vi "Initialize Amplitudes.vi"(0 "ToneCloud in":refnum<class "Tone Cloud.lvclass">, 5 "Level in":refnum<class "Level.lvclass">, 11 "error in (no error)":errorcluster) -> (4 "ToneCloud out":refnum<class "Tone Cloud.lvclass">, 15 "error out":errorcluster)   [LabVIEW 2020, in "Tone Cloud.lvclass"]
uses:
  Tone Cloud.lvclass
  Level/Level.lvclass
  Tone Cloud.lvclass/Tone Cloud.ctl
  Level/Level.lvclass/Level.ctl
  ce9a4e56-d8d9-4718-afa1-4568970c8e29.vi
  67dd2368-12ba-4959-8d3f-8fbbdd4b7264.vi
  595b4ae7-b8f7-4111-8c63-d399af629c05.vi
  Level/Read Units.vi
  Utility VIs/Math VIs/interp1 (2D).vi
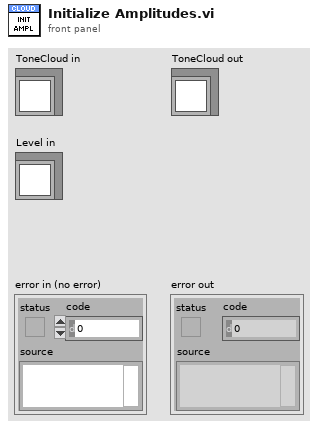
[diagram p1: front panel]
types:
  T1 = typedef "Level.lvclass/LevelUnits.ctl" = enum16{"dB atten", "dB SPL", "dB Vrms", "Volts", "dB mW", "mW", "dB HL", "dB SL"}
  T2 = typedef "Tone Cloud.lvclass/Level Mode.ctl" = enum16{"per component", "total rms"}
  T3 = cluster{"Freq (Hz)":dbl[], "Mag (dB SPL)":dbl[], "Phase (deg)":dbl[]}
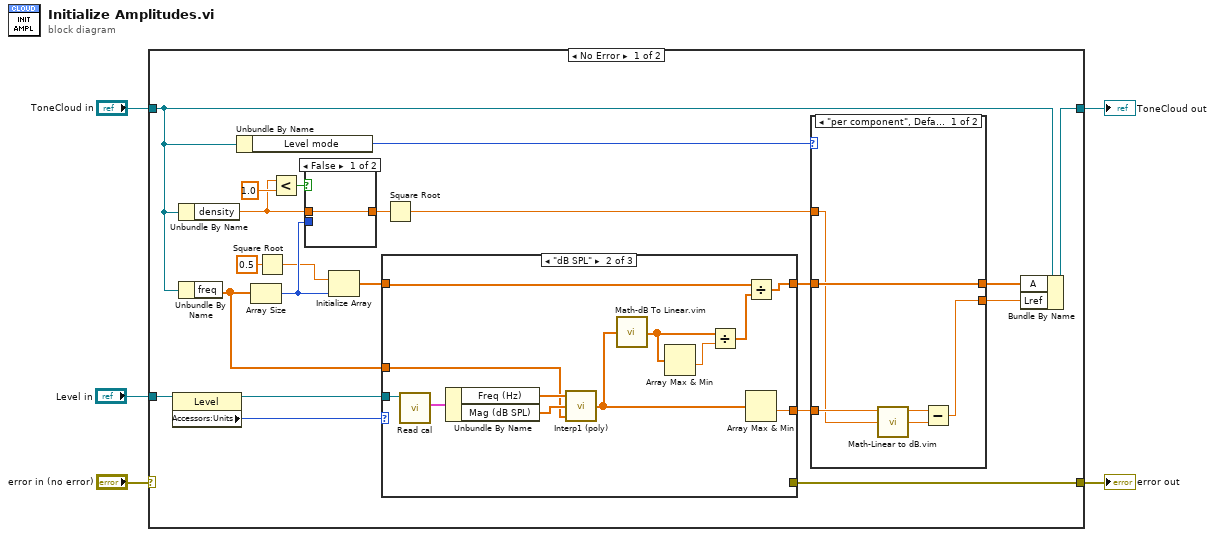
[diagram p0: block diagram]
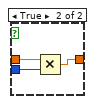
[diagram p2: hidden frame]
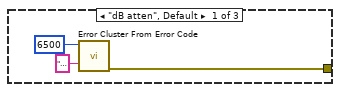
[diagram p3: hidden frame]
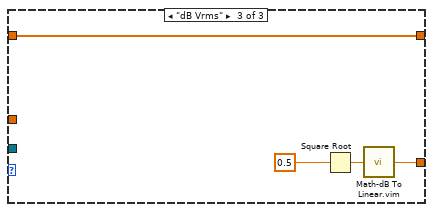
[diagram p4: hidden frame]
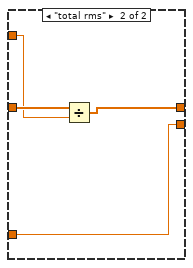
[diagram p5: hidden frame]
diagram:
  n1 = case shown="No Error" "error in (no error)" {
    selector: "error in (no error)" -> [_ w60]
    tunnel: [w22 w60] -> w4
    tunnel: [w24 w59] -> w2
    tunnel: "ToneCloud in" -> [w11 w59]
    tunnel: "Level in" -> [w26 _]
    frame No Error {
      n2 = property class="Level"(reference=w26) -> (reference out=w23:refnum<class "Level.lvclass">, "Accessors:Units"=w25:T1)  [unwired: 1 in, 1 out]
      n3 = Unbundle By Name(w11) -> ("density"=w20:dbl)
      n4 = Unbundle By Name(w11) -> ("freq"=w10:dbl[])
      n5 = Unbundle By Name(w11) -> ("Level mode"=w17:T2)
      n6 = Array Size(array=w10) -> (size(s)=w12:i32)
      n7 = Square Root(x=0.5) -> (sqrt(x)=w6:dbl)
      n8 = Less?(x=w20, y=1.0) -> (x < y?=w19:bool)
      n9 = case shown="False" w19 {
        tunnel: w20 -> [w27 w28]
        tunnel: [w27 w30] -> w18
        tunnel: w12 -> [_ w29]
        frame False {
        }
        frame True {
          n10 = Multiply(x=w28, y=w29) -> (x*y=w30:dbl)
        }
      }
      n11 = Initialize Array(w6, w12) -> (w8:dbl[])
      n12 = case shown="\"dB SPL\"" w25 {
        tunnel: w23 -> [_ w44 _]
        tunnel: [w31 _ _] -> w22
        tunnel: [_ w40 w46] -> w16
        tunnel: w10 -> [_ w41 _]
        tunnel: w8 -> [_ w39 w49]
        tunnel: [_ w38 w49] -> w7
        frame "dB atten", Default {
          n13 = call <vilib>:"Error Cluster From Error Code.vi"("error message (\"\")"="Tone Cloud level must be in units of dB SPL or dB Vrms" ("error message (\"\")"), "error code (0)"=6500) -> ("error out"=w31:errorcluster)  [unwired: 7 in]
        }
        frame "dB SPL" {
          n14 = call "Read cal.vi"("Level in"=w44) -> ("cal"=w45:T3)  [unwired: 8 in, 2 out]
          n15 = Unbundle By Name(w45) -> ("Freq (Hz)"=w43:dbl[], "Mag (dB SPL)"=w42:dbl[])
          n16 = call-poly "Interp1 (poly).vi"("X"=w43, "Y"=w42, "U"=w41) -> ("V"=w37:dbl[])  [unwired: 2 in]
          n17 = call "Math-dB To Linear.vim"("dB"=w37) -> ("linear"=w34:dbl[])
          n18 = Array Max & Min(array=w34) -> (min value=w36:dbl)  [unwired: 3 out]
          n19 = Divide(x=w34, y=w36) -> (x/y=w35:dbl[])
          n20 = Divide(x=w39, y=w35) -> (x/y=w38:dbl[])
          n21 = Array Max & Min(array=w37) -> (min value=w40:dbl)  [unwired: 3 out]
        }
        frame "dB Vrms" {
          n22 = Square Root(x=0.5) -> (sqrt(x)=w47:dbl)
          n23 = call "Math-dB To Linear.vim"("dB"=w47) -> ("linear"=w46:dbl)
        }
      }
      n24 = Square Root(x=w18) -> (sqrt(x)=w13:dbl)
      n25 = case shown="\"per component\", Default" w17 {
        tunnel: w13 -> [w50 w56]
        tunnel: w7 -> [w54 w57]
        tunnel: w16 -> [w53 w58]
        tunnel: [w54 w55] -> w15
        tunnel: [w52 w58] -> w14
        frame "per component", Default {
          n26 = call "Math-Linear to dB.vim"("linear"=w50) -> ("dB"=w51:dbl)
          n27 = Subtract(x=w53, y=w51) -> (x-y=w52:dbl)
        }
        frame "total rms" {
          n28 = Divide(x=w57, y=w56) -> (x/y=w55:dbl[])
        }
      }
      n29 = Bundle By Name(cluster=w11, "A"=w15, "Lref"=w14) -> (w24:refnum<class "Tone Cloud.lvclass">)
    }
    frame Error {
    }
  }
  "error out" <- w4
  "ToneCloud out" <- w2
